vi "Pre Launch Init.vi"(11 "客户端 in":refnum<class "客户端.lvclass"> caption="操作者输入") -> (0 "error out":errorcluster caption="错误输出", 3 "客户端 out":refnum<class "客户端.lvclass"> caption="操作者输出")   [LabVIEW 2015, in "客户端操作者.lvlib" / "客户端.lvclass"]
doc: "(<B>文件名</B>: Actor Framework.lvlib:Actor.lvclass:Pre Launch Init.vi)\n\n定义启动嵌套操作者方法被调用之后、操作者核心方法开始运行之前的操作。\n\n默认情况下，该方法不执行任何操作。子孙类重写该方法定义具体的操作。"
uses:
  <vilib>/ActorFramework/Actor/Actor.lvclass
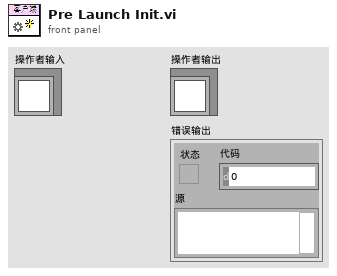
[diagram p1: front panel]
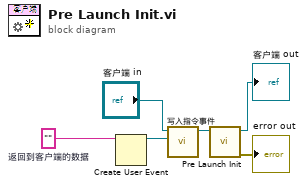
[diagram p0: block diagram]
diagram:
  w4 = ""  # 返回到客户端的数据
  n1 = Create User Event(user event datatype=w4) -> (user event=w3:refnum<user-event>)  [unwired: 1 in, 1 out]
  n2 = call-dynamic "写入指令事件.vi"("指令事件"=w3, "客户端输入"="客户端 in") -> ("客户端输出"=w1:refnum<class "客户端.lvclass">)  [unwired: 8 in, 1 out]
  n3 = call-parent "Pre Launch Init.vi"("Actor in"=w1) -> ("error out"=→"error out":errorcluster, "Actor out"=→"客户端 out":refnum<class "客户端.lvclass">)  [unwired: 9 in]
